vi "UpdateRender.vi"(6 "Instance":i32, 8 "error in (no error)":errorcluster) -> (0 "error out":errorcluster)   [LabVIEW 2017, in "PendulumLoop.lvlib"]
uses:
  PendulumLoop.lvlib
  Communication/Communication.lvlib
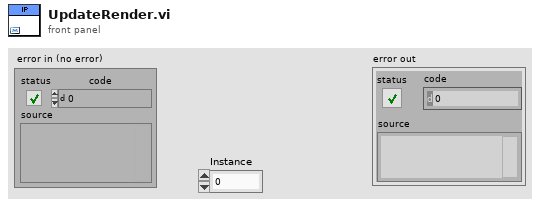
[diagram p1: front panel]
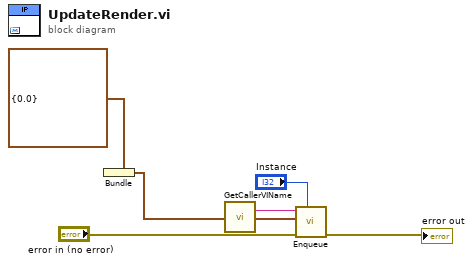
[diagram p0: block diagram]
diagram:
  n1 = Bundle(cluster=cluster{dbl} {0.0}) -> (w3:cluster{dbl})  [unwired: 1 in]
  n2 = call "GetCallerVIName.vi"() -> ("VI name"=w1:string)  [unwired: 11 in]
  n3 = call "Enqueue.vi"("Instance"="Instance", "error in (no error)"="error in (no error)", "Data"=w3, "Msg"=w1) -> ("error out"=→"error out":errorcluster)  [unwired: 7 in]
